vi "Speed Calculator.vi"(11 "stop":bool) -> ()   [LabVIEW 2014]
uses:
  <vilib>/rvi/interface/nirviOpenFPGA/nirviOpenFPGA.xnode
  <vilib>/rvi/interface/nirviCloseFPGA/nirviCloseFPGA.xnode
  <vilib>/rvi/interface/nirviReadWriteControl/nirviReadWriteControl.xnode
  <vilib>/Utility/error.llb/Error Cluster From Error Code.vi
  <vilib>/rvi/interface/Simulation/niFpgaSimulationCallBeginRW.vi
  <vilib>/rvi/errors/niLvFpgaAdjustHostInterfaceError.vi
  Global Data.vi
  FPGA Bitfiles/FormulaElectric2_FPGATarget_FPGA_FBcm5p3VDa4.lvbitx
  FPGA/Sensor Library/FPGA.vi
  <vilib>/FPGAPlugInAG/sbRIO-9626/niLvFpga_Open_sbRIO-9626.vi
  <vilib>/rvi/interface/common/dynamic/niFpgaDynamicAddResources.vi
  NiFpgaLv.dll
  <vilib>/FPGAPlugInAG/Dynamic/niLvFpga_Close_Dynamic.vi
panel:
  in  "Max Slip Time (ms)":u32=4000
  in  "Acceptable Speed Diff":dbl=0.05
  in  "Tire Diameter (m)":dbl=0.4064
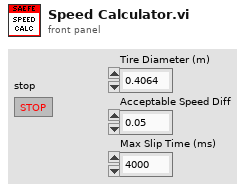
[diagram p1: front panel]
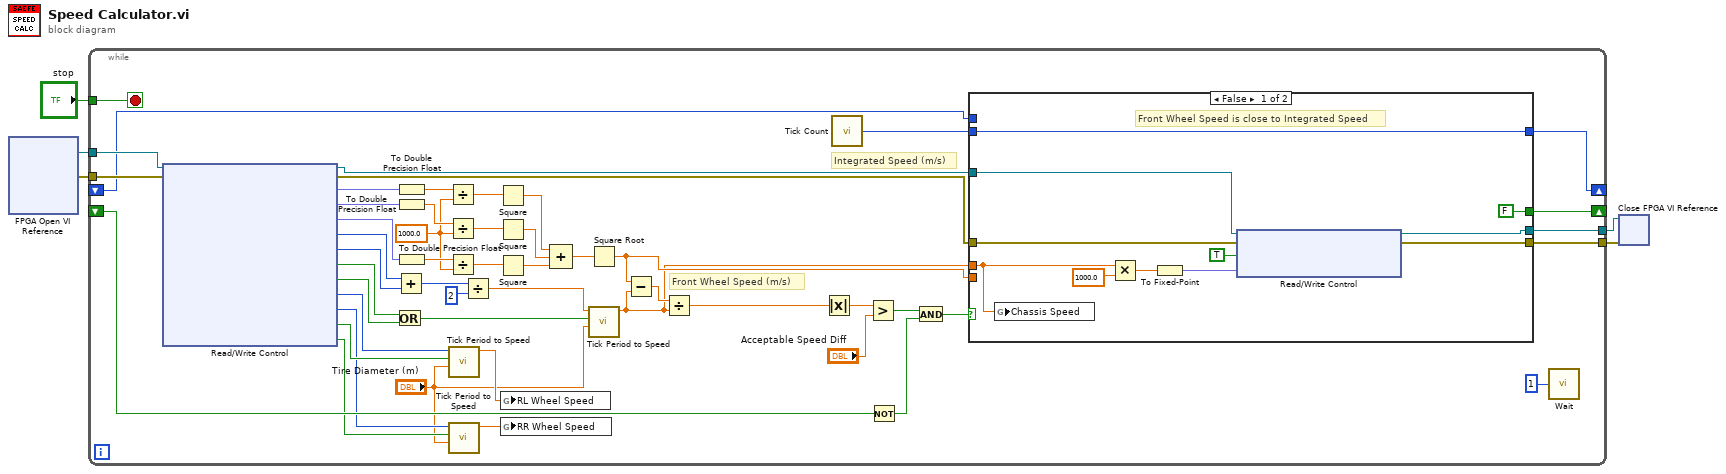
[diagram p0: block diagram]
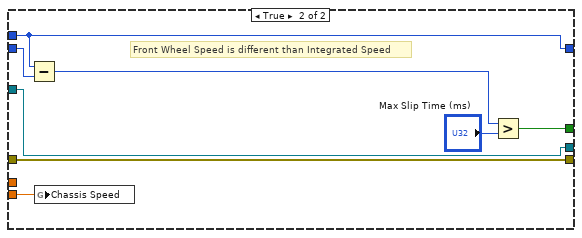
[diagram p2: hidden frame]
diagram:
  n1 = xnode "FPGA Open VI Reference"() -> ("FPGA VI Reference Out"=w4:refnum<k20>, "error out"=w3:errorcluster)  [unwired: 2 in]
  n2 = while {
    tunnel: "stop" -> [w56]
    tunnel: w4 -> [w54]
    tunnel: w3 -> [w53]
    tunnel: [w29] -> w2
    tunnel: [w27] -> w1
    shift-right: [w25] -> _
    shift-left: _ -> [w24]
    shift-right: [w23] -> _
    shift-left: _ -> [w18]
    stop <- w56 stop-if-true
    w46 = 1000.0 ("y")
    # "Integrated Speed (m/s)"
    # "Front Wheel Speed (m/s)"
    n3 = xnode "Read/Write Control"("FPGA VI Reference In"=w54, "error in"=w53) -> ("FPGA VI Reference Out"=w30:refnum<k20>, "error out"=w28:errorcluster, "Integrated SpeedX (m/s )*(us)"=w52:fxp<+/-,32,29>, "Integrated SpeedY"=w51:fxp<+/-,32,29>, "Integrated SpeedZ"=w50:fxp<+/-,32,29>, "FL Tick Period"=w38:u32, "FR Tick Period"=w37:u32, "FL Stopped"=w16:bool, "FR Stopped"=w15:bool, "RL Tick Period"=w12:u32, "RR Tick Period"=w9:u32, "RL Stopped"=w11:bool, "RR Stopped"=w8:bool)
    n4 = Or(x=w16, y=w15) -> (x .or. y?=w14:bool)
    n5 = Add(x=w38, y=w37) -> (x+y=w36:u32)
    n6 = To Double Precision Float(number=w52) -> (double precision float=w49:dbl)
    n7 = To Double Precision Float(number=w51) -> (double precision float=w48:dbl)
    n8 = To Double Precision Float(number=w50) -> (double precision float=w47:dbl)
    n9 = Divide(x=w49, y=w46) -> (x/y=w45:dbl)
    n10 = Divide(x=w48, y=w46) -> (x/y=w43:dbl)
    n11 = Divide(x=w47, y=w46) -> (x/y=w44:dbl)
    n12 = call "Tick Period to Speed.vi"("Tire Diameter (m)"="Tire Diameter (m)", "Boolean"=w11, "Tick Period"=w12) -> ("Wheel Speed (m/s)"=w10:dbl)  [unwired: 8 in]
    n13 = call "Tick Period to Speed.vi"("Tire Diameter (m)"="Tire Diameter (m)", "Boolean"=w8, "Tick Period"=w9) -> ("Wheel Speed (m/s)"=w6:dbl)  [unwired: 8 in]
    n14 = Divide(x=w36, y=u32 2) -> (x/y=w13:dbl)
    n15 = Square(x=w45) -> (x^2=w41:dbl)
    n16 = Square(x=w43) -> (x^2=w42:dbl)
    n17 = Square(x=w44) -> (x^2=w40:dbl)
    n18 = global write "Global Data.vi" "RL Wheel Speed"(w10) -> ()
    n19 = global write "Global Data.vi" "RR Wheel Speed"(w6) -> ()
    n20 = Compound Arithmetic op=unknown(w41, w42, w40) -> (w39:dbl)
    n21 = Square Root(x=w39) -> (sqrt(x)=w34:dbl)
    n22 = call "Tick Period to Speed.vi"("Tire Diameter (m)"="Tire Diameter (m)", "Boolean"=w14, "Tick Period"=w13) -> ("Wheel Speed (m/s)"=w32:dbl)  [unwired: 8 in]
    n23 = Subtract(x=w34, y=w32) -> (x-y=w33:dbl)
    n24 = Divide(x=w33, y=w32) -> (x/y=w21:dbl)
    n25 = Absolute Value(x=w21) -> (abs(x)=w22:dbl)
    n26 = call "Tick Count"() -> ("Tick Count(mSec)"=w26:u32)
    n27 = Greater?(x=w22, y="Acceptable Speed Diff") -> (0:w20:bool)
    n28 = Not(x=w18) -> (.not. x?=w19:bool)
    n29 = And(x=w20, y=w19) -> (x .and. y?=w17:bool)
    n30 = case shown="False" w17 {
      tunnel: w34 -> [_ w73]
      tunnel: w32 -> [w59 _]
      tunnel: w30 -> [w67 w75]
      tunnel: [w66 w75] -> w29
      tunnel: w28 -> [w65 w74]
      tunnel: [w64 w74] -> w27
      tunnel: w26 -> [w58 w71]
      tunnel: [w58 w72] -> w25
      tunnel: w24 -> [_ w72]
      tunnel: [FALSE w68] -> w23
      frame False {
        # "Front Wheel Speed is close to Integrated Speed"
        n31 = global write "Global Data.vi" "Chassis Speed"(w59) -> ()
        n32 = Multiply(x=w59, y=1000.0) -> (x*y=w61:dbl)
        n33 = To Fixed-Point(number=w61) -> (fixed-point=w62:fxp<+/-,32,29>)  [unwired: 1 in]
        n34 = xnode "Read/Write Control"("FPGA VI Reference In"=w67, "error in"=w65, "Reset Speed"=TRUE, "Reset Integrated Speed To..."=w62) -> ("FPGA VI Reference Out"=w66:refnum<k20>, "error out"=w64:errorcluster)
      }
      frame True {
        # "Front Wheel Speed is different than Integrated Speed"
        n35 = Subtract(x=w72, y=w71) -> (x-y=w70:u32)
        n36 = global write "Global Data.vi" "Chassis Speed"(w73) -> ()
        n37 = Greater?(x=w70, y="Max Slip Time (ms)") -> (0:w68:bool)
      }
    }
    n38 = call "Wait"("Count(mSec)"=u32 1) -> ()  [unwired: 1 out]
  }
  n39 = xnode "Close FPGA VI Reference"("FPGA VI Reference In"=w2, "error in"=w1) -> ()  [unwired: 1 out]
